vi "PSO_Rank Population.vi"(11 "Population in":T1) -> (3 "Population out":T1)   [LabVIEW 2016, in "Optimal Frequency Bands Search.lvlib" / "ParticleSwarm.lvlib"]
doc: "Ранжирование особей популяции в зависимости от значения функции приспособленности"
uses:
  ParticleSwarm.lvlib
  PSO_tPopulation.ctl
panel:
  # "This VI is a part of BCI Design library, http://www.ru-bci.org \nCopyright © 2020, Sotnikov Peter, All rights reserved. License: GNU GPLv3"
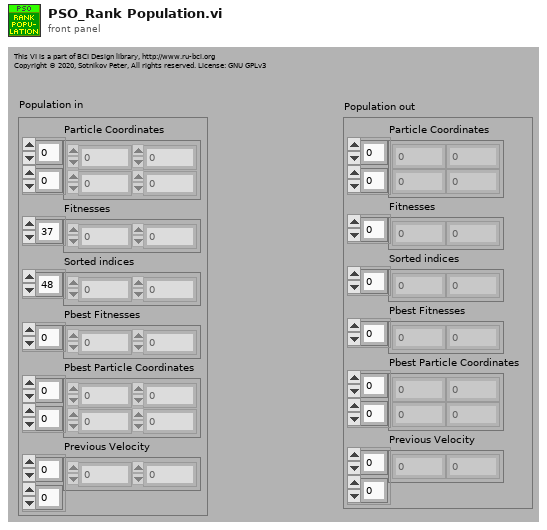
[diagram p1: front panel]
types:
  T1 = typedef "Optimal Frequency Bands Search.lvlib/ParticleSwarm.lvlib/PSO_tPopulation.ctl" = cluster{"Particle Coordinates":i32[][], "Fitnesses":dbl[], "Sorted indices":i32[], "Pbest Fitnesses":dbl[], "Pbest Particle Coordinates":i32[][], "Previous Velocity":dbl[][]}
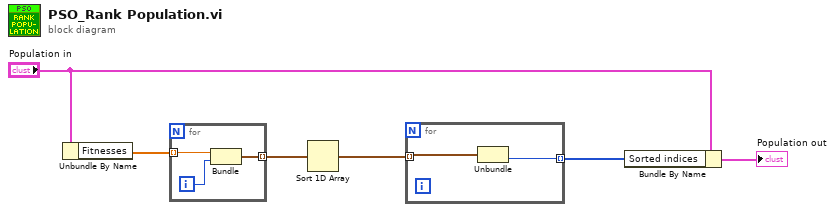
[diagram p0: block diagram]
diagram:
  n1 = Unbundle By Name("Population in") -> ("Fitnesses"=w4:dbl[])
  n2 = for {
    tunnel: w4 -> [w9] mode=indexing
    tunnel: [w7] -> w6 mode=indexing
    i -> [w8]
    n3 = Bundle("Numeric"=w9, w8) -> (w7:cluster{"Numeric":dbl, i32})  [unwired: 1 in]
  }
  n4 = Sort 1D Array(array=w6) -> (sorted array=w5:cluster{"Numeric":dbl, i32}[])
  n5 = for {
    tunnel: w5 -> [w11] mode=indexing
    tunnel: [w10] -> w2 mode=indexing
    n6 = Unbundle(w11) -> (w10:i32)  [unwired: 1 out]
  }
  n7 = Bundle By Name(cluster="Population in", "Sorted indices"=w2) -> (→"Population out":T1)
